vi "RTS Custom Command Parse.vi"(8 "Error In":errorcluster, 11 "Input String":string) -> (0 "Error Out":errorcluster, 1 "Register to Write":i32, 2 "Address":i32, 3 "Clean Input String":string)   [LabVIEW 2016]
uses:
  <vilib>/Utility/error.llb/whitespace.ctl
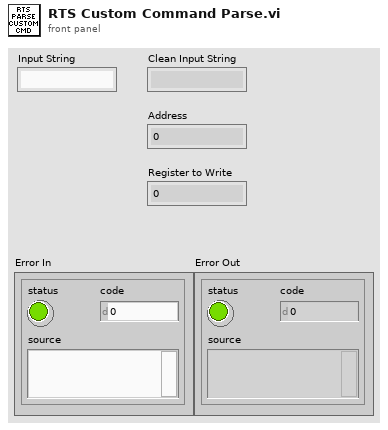
[diagram p1: front panel]
types:
  T1 = typedef "whitespace.ctl" = u16
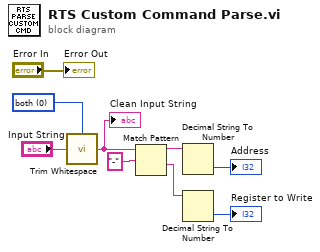
[diagram p0: block diagram]
diagram:
  w5 = T1 0 items=["both", "start of string", "end of string"] ("location (both)")
  n1 = call <vilib>:"Trim Whitespace.vi"("string"="Input String", "location (both)"=w5) -> ("trimmed string"=w4:string)
  "Clean Input String" <- w4
  n2 = Match Pattern(string=w4, regular expression="-") -> (before substring=w6:string, after substring=w7:string)  [unwired: 1 in, 2 out]
  n3 = Decimal String To Number(string=w6) -> (number=→"Address":i32)  [unwired: 2 in, 1 out]
  n4 = Decimal String To Number(string=w7) -> (number=→"Register to Write":i32)  [unwired: 2 in, 1 out]
  "Error Out" <- "Error In"
